vi "Open Project.vi"(7 "Open Project Window ?":bool, 8 "error in (no error)":errorcluster, 10 "Project Path in":path, 11 "Application reference":refnum<vi>) -> (0 "error out":errorcluster, 2 "Project out":refnum<vi>, 3 "Application out":refnum<vi>)   [LabVIEW 2019, in "gRPC Scripting Tools.lvlib"]
uses:
  gRPC Scripting Tools.lvlib
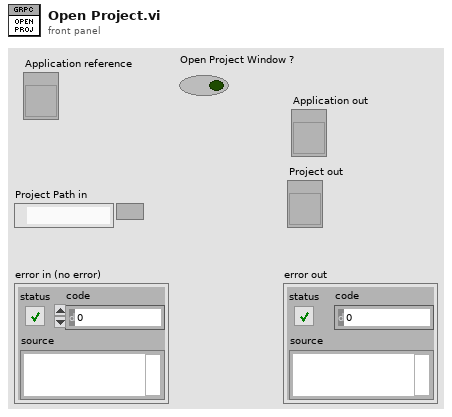
[diagram p1: front panel]
types:
  T1 = enum32{"invalid app kind", "Development System", "Run Time System", "Student Edition", "Embedded LabVIEW", "Evaluation", "Custom"}
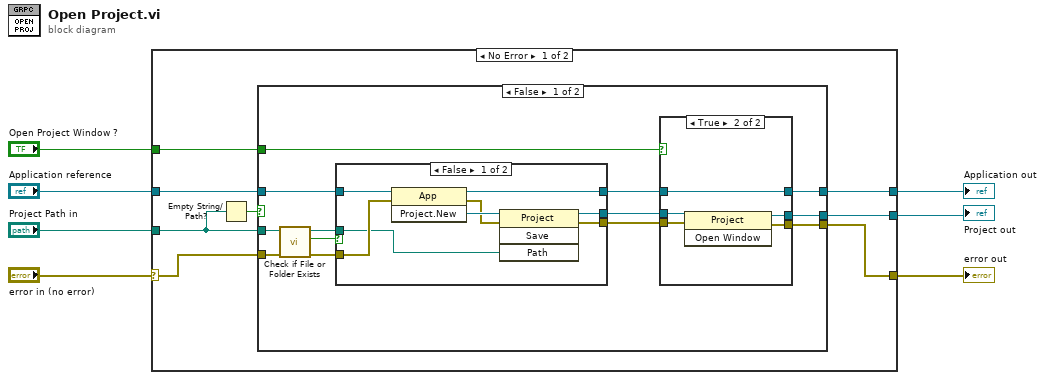
[diagram p0: block diagram]
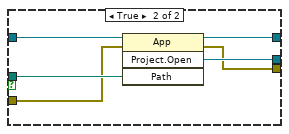
[diagram p3: hidden frame]
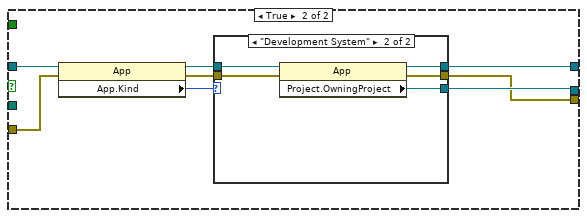
[diagram p4: hidden frame]
diagram:
  n1 = case shown="No Error" "error in (no error)" {
    selector: "error in (no error)" -> [w13 w66]
    tunnel: "Project Path in" -> [w10 _]
    tunnel: [w12 _] -> w6
    tunnel: "Open Project Window ?" -> [w11 _]
    tunnel: [w15 _] -> w4
    tunnel: [w14 w66] -> w3
    tunnel: "Application reference" -> [w8 _]
    frame No Error {
      n2 = Empty String/Path?(string/path=w10) -> (empty?=w9:bool)
      n3 = case shown="False" w9 {
        tunnel: w10 -> [w28 _]
        tunnel: [w22 w57] -> w15
        tunnel: [w21 w56] -> w14
        tunnel: w13 -> [w20 w53]
        tunnel: [w18 w58] -> w12
        tunnel: w11 -> [w17 _]
        tunnel: w8 -> [w16 w51]
        frame False {
          n4 = call <vilib>:"Check if File or Folder Exists.vi"("error in (no error)"=w20, "path"=w28) -> ("error out"=w25:errorcluster, "file or folder exists?"=w26:bool, "dup path"=w27:path)  [unwired: 7 in]
          n5 = case shown="False" w26 {
            tunnel: [w39 w47] -> w24
            tunnel: w27 -> [w40 w50]
            tunnel: w25 -> [w43 w48]
            tunnel: [w41 w49] -> w19
            tunnel: [w38 w46] -> w23
            tunnel: w16 -> [w37 w45]
            frame False {
              n6 = invoke class="App" method="Project.New"(reference=w37, error in=w43) -> (reference out=w41:refnum<vi>, error out=w42:errorcluster, "Project:New"=w44:refnum<vi>)  [unwired: 1 in]
              n7 = invoke class="Project" method="Save"(reference=w44, error in=w42, "Path"=w40) -> (reference out=w39:refnum<vi>, error out=w38:errorcluster)  [unwired: 1 in, 2 out]
            }
            frame True {
              n8 = invoke class="App" method="Project.Open"(reference=w45, error in=w48, "Path"=w50) -> (reference out=w49:refnum<vi>, error out=w46:errorcluster, "Project:Open"=w47:refnum<vi>)  [unwired: 1 in, 1 out]
            }
          }
          n9 = case shown="True" w17 {
            tunnel: w24 -> [w30 w36]
            tunnel: w23 -> [w29 w35]
            tunnel: [w30 w34] -> w22
            tunnel: [w29 w33] -> w21
            tunnel: w19 -> [w31 w32]
            tunnel: [w31 w32] -> w18
            frame False {
            }
            frame True {
              n10 = invoke class="Project" method="Open Window"(reference=w36, error in=w35) -> (reference out=w34:refnum<vi>, error out=w33:errorcluster)  [unwired: 1 in, 1 out]
            }
          }
        }
        frame True {
          n11 = property class="App"(reference=w51, error in=w53) -> (reference out=w54:refnum<vi>, error out=w52:errorcluster, "App.Kind"=w55:T1)
          n12 = case shown="\"Development System\"" w55 {
            tunnel: [w60 w65] -> w58
            tunnel: [_ w64] -> w57
            tunnel: [w59 w63] -> w56
            tunnel: w54 -> [w60 w62]
            tunnel: w52 -> [w59 w61]
            frame "invalid app kind", Default {
            }
            frame "Development System" {
              n13 = property class="App"(reference=w62, error in=w61) -> (reference out=w65:refnum<vi>, error out=w63:errorcluster, "Project.OwningProject"=w64:refnum<vi>)
            }
          }
        }
      }
    }
    frame Error {
    }
  }
  "Project out" <- w4
  "error out" <- w3
  "Application out" <- w6
